vi "_Get Startup Folder.vi"(1 "FileName":string="Config") -> (0 "FilePath":path)   [LabVIEW 2012]
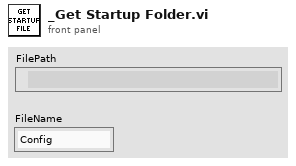
[diagram p1: front panel]
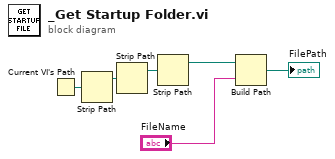
[diagram p0: block diagram]
diagram:
  n1 = Current VI's Path() -> (path=w4:path)
  n2 = Strip Path(path=w4) -> (stripped path=w5:path)  [unwired: 1 out]
  n3 = Strip Path(path=w5) -> (stripped path=w6:path)  [unwired: 1 out]
  n4 = Strip Path(path=w6) -> (stripped path=w2:path)  [unwired: 1 out]
  n5 = Build Path(base path=w2, name or relative path="FileName") -> (appended path=→"FilePath":path)
